vi "Close.vi"(8 "error in (no error)":errorcluster, 11 "VISA resource name":refnum<visa-resource-name>) -> (0 "error out":errorcluster)   [LabVIEW 2020, in "HandsOnPi2040.lvlib"]
doc: "Performs an instrument error query before terminating the software connection to the instrument."
uses:
  HandsOnPi2040.lvlib
panel:
  # "Input"
  # "Output"
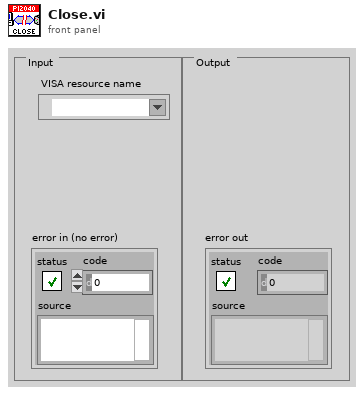
[diagram p1: front panel]
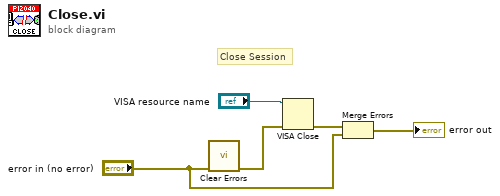
[diagram p0: block diagram]
diagram:
  # "Close Session"
  n1 = call <vilib>:"Clear Errors.vi"("error in (no error)"="error in (no error)") -> ("error out"=w4:errorcluster)  [unwired: 5 in, 1 out]
  n2 = VISA Close(VISA resource name="VISA resource name", error in (no error)=w4) -> (error out=w5:errorcluster)
  n3 = Merge Errors(w5, "error in (no error)") -> (→"error out":errorcluster)
